vi "Spin echo.vi"(0 "Free precession time":dbl[unit], 1 "MW switch margin (ns)":dbl, 2 "resolution (ns)":dbl, 5 "margin (ns)":i32, 7 "Gain":dbl, 9 "pi":dbl[unit], 12 "AOM on":dbl[unit], 13 "AOM off":dbl[unit], 14 "pi/2":dbl[unit]) -> (4 "Array size":i32, 6 "I":dbl[](array[numeric]), 8 "Q":dbl[](array[numeric]))   [LabVIEW 2015]
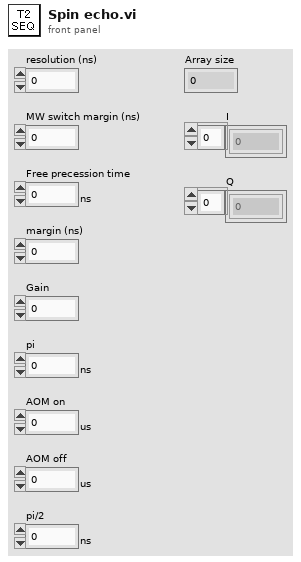
[diagram p1: front panel]
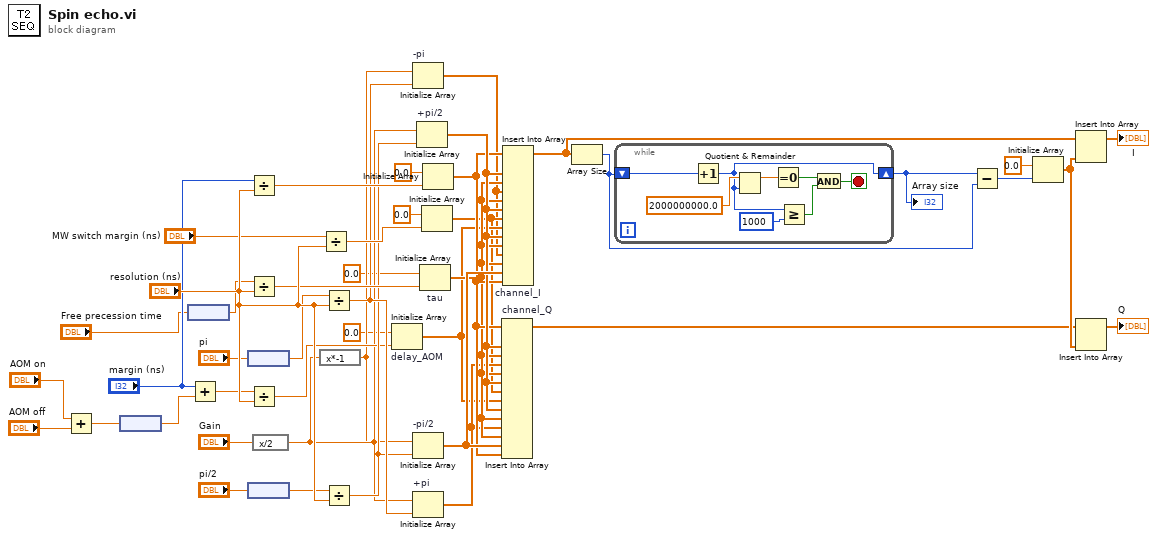
[diagram p0: block diagram]
diagram:
  n1 = Add(x="AOM on", y="AOM off") -> (x+y=w9:dbl[unit])
  n2 = node(w9) -> (w13:dbl)
  n3 = node("Free precession time") -> (w37:dbl)
  n4 = Add(x="margin (ns)", y=w13) -> (x+y=w30:dbl)
  n5 = node("pi") -> (w34:dbl)
  n6 = node("pi/2") -> (w32:dbl)
  n7 = Divide(x="margin (ns)", y="resolution (ns)") -> (x/y=w39:dbl)
  n8 = Divide(x=w37, y="resolution (ns)") -> (x/y=w36:dbl)
  n9 = Divide(x=w30, y="resolution (ns)") -> (x/y=w31:dbl)
  n10 = expression code="x/2"("Gain") -> (w27:dbl)
  n11 = expression code="x*-1"(w27) -> (w26:dbl)
  n12 = Divide(x="MW switch margin (ns)", y="resolution (ns)") -> (x/y=w41:dbl)
  n13 = Divide(x=w34, y="resolution (ns)") -> (x/y=w35:dbl)
  n14 = Divide(x=w32, y="resolution (ns)") -> (x/y=w33:dbl)
  n15 = Initialize Array "delay_AOM"(0.0 ("element"), w31) -> (w15:dbl[])
  n16 = Initialize Array "-pi"(w26, w35) -> (w12:dbl[])
  n17 = Initialize Array "-pi/2"(w26, w33) -> (w29:dbl[])
  n18 = Initialize Array "+pi"(w27, w35) -> (w16:dbl[])
  n19 = Initialize Array "+pi/2"(w27, w33) -> (w28:dbl[])
  n20 = Initialize Array "tau"(0.0 ("element"), w36) -> (w17:dbl[])
  n21 = Initialize Array(0.0 ("element"), w41) -> (w14:dbl[])
  n22 = Initialize Array(0.0 ("element"), w39) -> (w18:dbl[])
  n23 = Insert Into Array "channel_Q"(array=w18, new element #1=w28, new element #2=w17, new element #3=w16, new element #4=w17, new element #5=w28, new element #6=w14, new element #7=w15, new element #8=w28, new element #9=w17, new element #10=w16, new element #11=w17, new element #12=w29, new element #13=w18) -> (w23:dbl[])  [unwired: 1 in]
  n24 = Insert Into Array "channel_I"(array=w18, new element #1=w28, new element #2=w17, new element #3=w12, new element #4=w17, new element #5=w28, new element #6=w14, new element #7=w15, new element #8=w28, new element #9=w17, new element #10=w12, new element #11=w17, new element #12=w29, new element #13=w18) -> (w21:dbl[])  [unwired: 1 in]
  n25 = Array Size(array=w21) -> (size(s)=w43:i32)
  n26 = while {
    shift-right: [w46] -> w44
    shift-left: w43 -> [w52]
    stop <- w48 stop-if-true
    n27 = Increment(x=w52) -> (x+1=w46:i32)
    n28 = Quotient & Remainder(x=2000000000.0, y=w46) -> (x-y*floor(x/y)=w50:dbl)  [unwired: 1 out]
    n29 = Equal To 0?(x=w50) -> (x = 0?=w47:bool)
    n30 = Greater Or Equal?(x=w46, y=1000) -> (x >= y?=w49:bool)
    n31 = And(x=w47, y=w49) -> (x .and. y?=w48:bool)
  }
  "Array size" <- w44
  n32 = Subtract(x=w44, y=w43) -> (x-y=w19:i32)
  n33 = Initialize Array(0.0 ("element"), w19) -> (w24:dbl[])
  n34 = Insert Into Array(array=w21, new element=w24) -> (→"I":dbl[])  [unwired: 1 in]
  n35 = Insert Into Array(array=w23, new element=w24) -> (→"Q":dbl[])  [unwired: 1 in]
